vi "DefineTankBoundaries.vi"(7 "tank_resolution":T3, 8 "error in (no error)":errorcluster, 9 "liquid":T1={"liquid_temperature"=array75x50[3750 elements], "water_level"=1.4948979591836733, "room_temperature"=298.15}, 10 "heater":T2={"heater_width"=0.5, "heater_heat"=50.0}, 11 "PDE in":refnum<class "NI_PDE.lvclass">) -> (0 "error out":errorcluster, 3 "PDE out":refnum<class "NI_PDE.lvclass">)   [LabVIEW 2020]
uses:
  <vilib>/gmath/pde.llb/PDEClass/NI_PDE.lvclass
  TankResolution.ctl
  Heater.ctl
  Liquid.ctl
  <vilib>/gmath/pde.llb/Common/PDE_BC Type.ctl
  <vilib>/gmath/pde.llb/Common/PDE_BC Position 2D.ctl
  <vilib>/gmath/pde.llb/Define 2D Heat PDE BC (Numeric).vi
  <vilib>/gmath/NI_PDE.lvlib
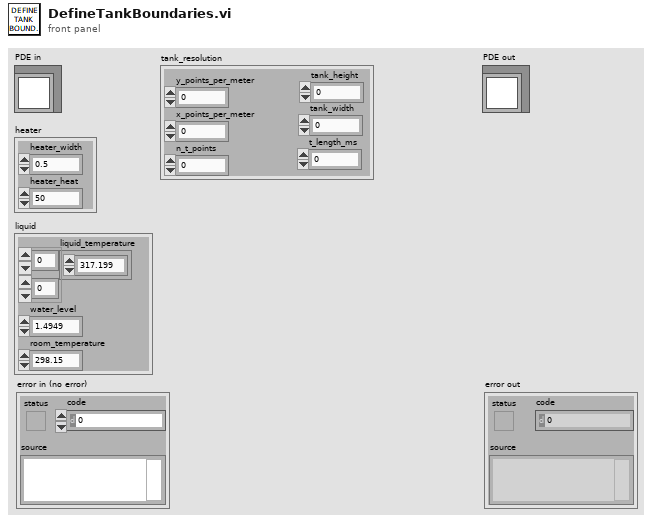
[diagram p1: front panel]
types:
  T1 = typedef "Liquid.ctl" = cluster{"liquid_temperature":dbl[][], "water_level":dbl, "room_temperature":dbl}
  T2 = typedef "Heater.ctl" = cluster{"heater_width":dbl, "heater_heat":dbl}
  T3 = typedef "TankResolution.ctl" = cluster{"y_points_per_meter":i32, "x_points_per_meter":i32, "n_t_points":i32, "tank_height":dbl, "tank_width":dbl, "t_length_ms":u32}
  T4 = typedef "NI_PDE.lvlib/PDE_BC Position 2D.ctl" = i32
  T5 = typedef "NI_PDE.lvlib/PDE_BC Type.ctl" = i32
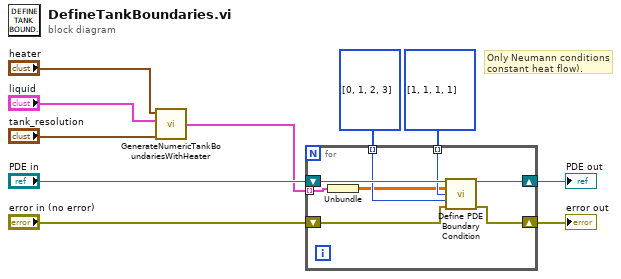
[diagram p0: block diagram]
diagram:
  w8 = T4[] [0, 1, 2, 3] items=["Start X", "End X", "Start Y", "End Y"]
  w3 = T5[] [1, 1, 1, 1] items=["Dirichlet", "Neumann"]
  # "Only Neumann conditions \nconstant heat flow)."
  n1 = call "GenerateNumericTankBoundariesWithHeater.vi"("tank_resolution"="tank_resolution", "liquid"="liquid", "heater"="heater") -> ("numeric_boundaries"=w7:cluster{dbl[][]}[])  [unwired: 3 in]
  n2 = for {
    shift-right: [w14] -> w6
    shift-left: "PDE in" -> [w18]
    shift-right: [w13] -> w5
    shift-left: "error in (no error)" -> [w17]
    tunnel: w8 -> [w16] mode=indexing
    tunnel: w3 -> [w15] mode=indexing
    tunnel: w7 -> [w12] mode=indexing
    n3 = Unbundle(w12) -> (w11:dbl[][])
    n4 = call-poly <vilib>:"Define PDE Boundary Condition.vi"("PDE in"=w18, "Boundary Condition"=w11, "type"=w15, "position"=w16, "error in (no error)"=w17) -> ("PDE out"=w14:refnum<class "NI_PDE.lvclass">, "error out"=w13:errorcluster)  [unwired: 9 in]
  }
  "PDE out" <- w6
  "error out" <- w5
